vi "Init with SQL Records.vi"(8 "error in (no error)":errorcluster, 10 "SQL Dataset":variant[][](array[variant]), 11 "Statement in":refnum<class "TransactionList.lvclass">) -> (0 "error out":errorcluster, 3 "Statement out":refnum<class "TransactionList.lvclass">)   [LabVIEW 2018, in "TransactionList.lvclass"]
uses:
  TransactionList.lvclass
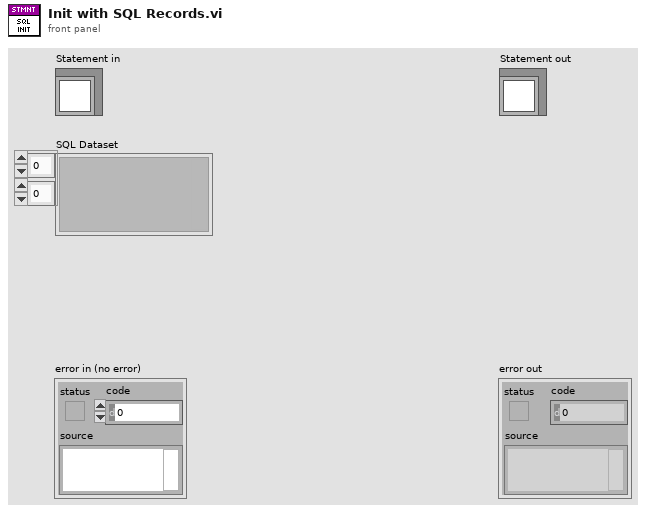
[diagram p1: front panel]
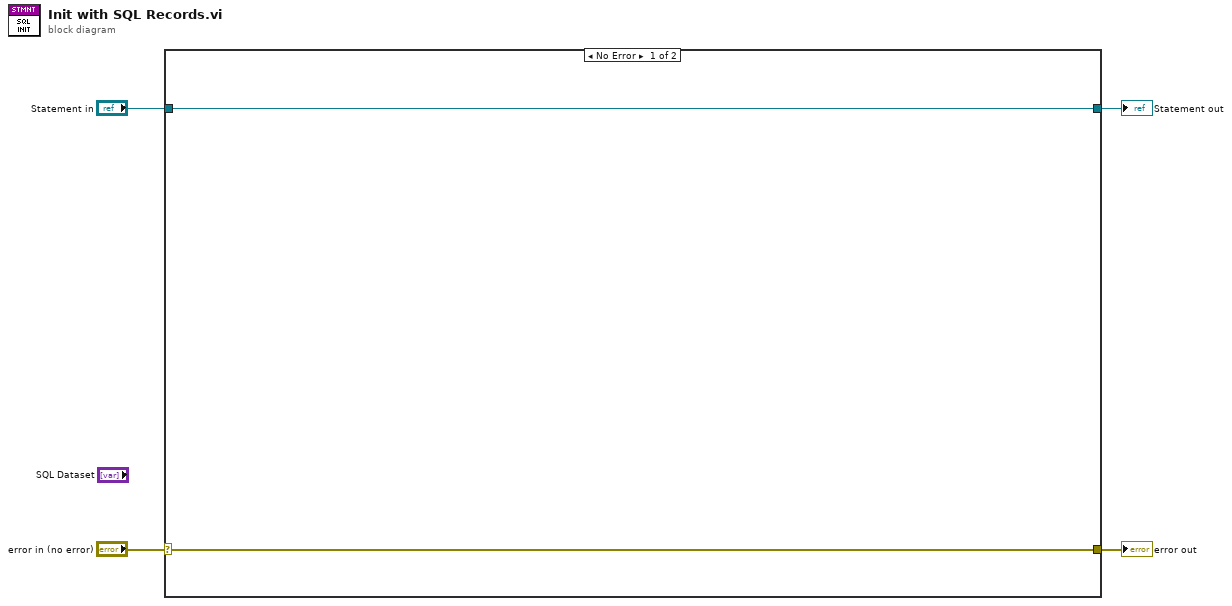
[diagram p0: block diagram]
diagram:
  n1 = case shown="No Error" "error in (no error)" {
    selector: "error in (no error)" -> [w6 w8]
    tunnel: [w6 w8] -> w3
    tunnel: [w5 w7] -> w1
    tunnel: "Statement in" -> [w5 w7]
    frame No Error {
    }
    frame Error {
    }
  }
  "error out" <- w3
  "Statement out" <- w1
